vi "RTS Post Client Setup Data.vi"(8 "Error In":errorcluster, 10 "File Setup Data":string[][](array[string]), 11 "Station Settings In":T1) -> (0 "Error Out":errorcluster, 3 "Station Settings Out":T1)   [LabVIEW 2016]
uses:
  Type Definitions/RTS Station Settions TCP Comms.ctl
  Type Definitions/RTS Chamber Save Status.ctl
  Type Definitions/RTS Test Pattern.ctl
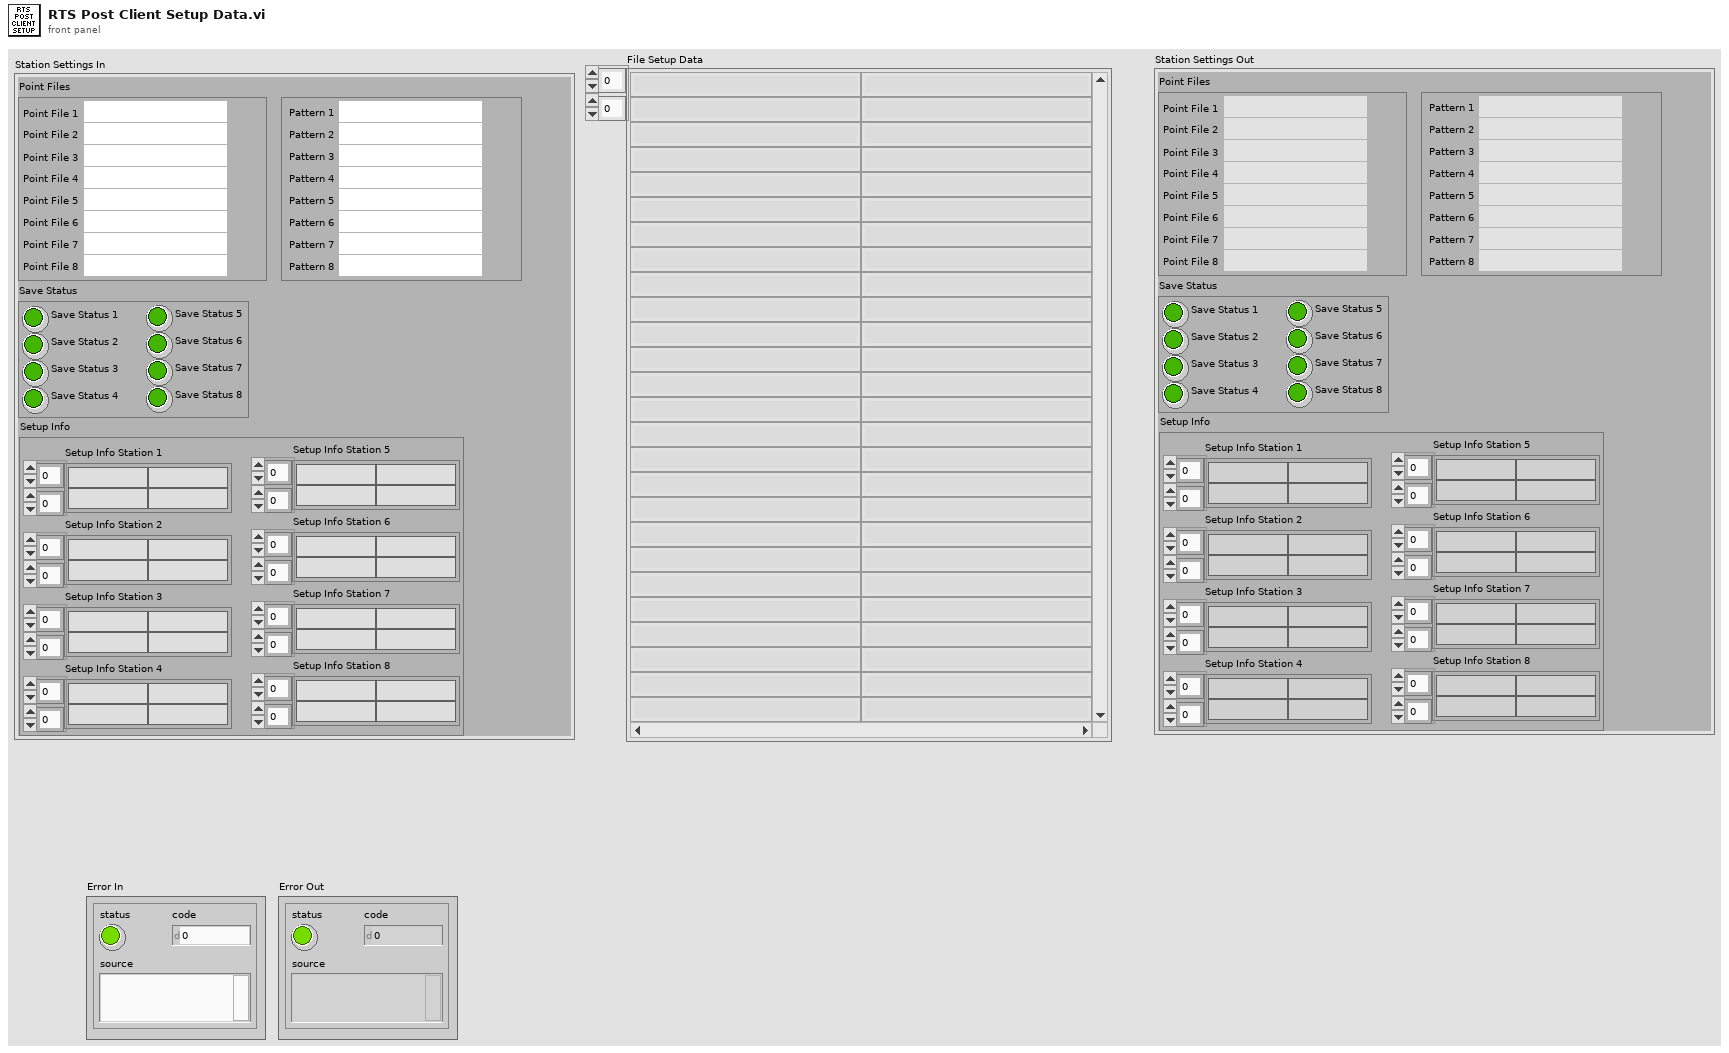
[diagram p1: front panel]
types:
  T1 = typedef "RTS Station Settions TCP Comms.ctl" = cluster{"Point Files":cluster{"Point File 1":path, "Point File 2":path, "Point File 3":path, "Point File 4":path, "Point File 5":path, "Point File 6":path, "Point File 7":path, "Point File 8":path}, "Save Status":T2, "Setup Info":cluster{"Setup Info Station 1":string[][], "Setup Info Station 2":string[][], "Setup Info Station 3":string[][], "Setup Info Station 4":string[][], "Setup Info Station 5":string[][], "Setup Info Station 6":string[][], "Setup Info Station 7":string[][], "Setup Info Station 8":string[][]}, "Chamber Test Pattern":T3}
  T2 = typedef "RTS Chamber Save Status.ctl" = cluster{"Save Status 1":bool, "Save Status 2":bool, "Save Status 3":bool, "Save Status 4":bool, "Save Status 5":bool, "Save Status 6":bool, "Save Status 7":bool, "Save Status 8":bool}
  T3 = typedef "RTS Test Pattern.ctl" = cluster{" Pattern 1":path, "Pattern 2":path, "Pattern 3":path, "Pattern 4":path, "Pattern 5":path, "Pattern 6":path, "Pattern 7":path, "Pattern 8":path}
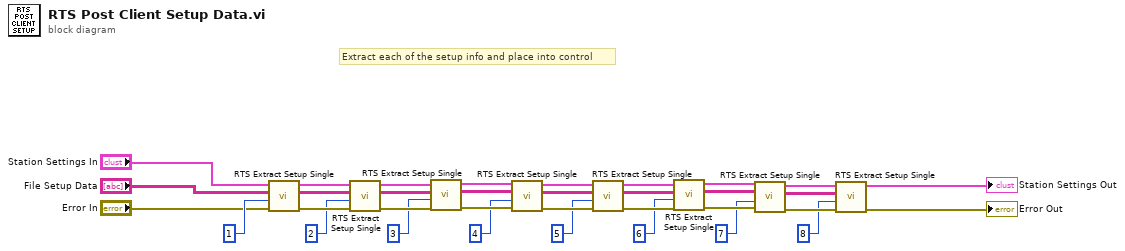
[diagram p0: block diagram]
diagram:
  # "Extract each of the setup info and place into control"
  n1 = call "RTS Extract Setup Single.vi"("Error In"="Error In", "Station Number"=u8 1, "File Setup Data"="File Setup Data", "Station Settings In in"="Station Settings In") -> ("Error Out"=w29:errorcluster, "Updated Array"=w31:string[][], "Station Settings In out"=w30:T1)  [unwired: 5 in]
  n2 = call "RTS Extract Setup Single.vi"("Error In"=w29, "Station Number"=u8 2, "File Setup Data"=w31, "Station Settings In in"=w30) -> ("Error Out"=w28:errorcluster, "Updated Array"=w22:string[][], "Station Settings In out"=w15:T1)  [unwired: 5 in]
  n3 = call "RTS Extract Setup Single.vi"("Error In"=w28, "Station Number"=u8 3, "File Setup Data"=w22, "Station Settings In in"=w15) -> ("Error Out"=w27:errorcluster, "Updated Array"=w21:string[][], "Station Settings In out"=w14:T1)  [unwired: 5 in]
  n4 = call "RTS Extract Setup Single.vi"("Error In"=w27, "Station Number"=u8 4, "File Setup Data"=w21, "Station Settings In in"=w14) -> ("Error Out"=w26:errorcluster, "Updated Array"=w20:string[][], "Station Settings In out"=w13:T1)  [unwired: 5 in]
  n5 = call "RTS Extract Setup Single.vi"("Error In"=w26, "Station Number"=u8 5, "File Setup Data"=w20, "Station Settings In in"=w13) -> ("Error Out"=w25:errorcluster, "Updated Array"=w19:string[][], "Station Settings In out"=w12:T1)  [unwired: 5 in]
  n6 = call "RTS Extract Setup Single.vi"("Error In"=w25, "Station Number"=u8 6, "File Setup Data"=w19, "Station Settings In in"=w12) -> ("Error Out"=w24:errorcluster, "Updated Array"=w18:string[][], "Station Settings In out"=w11:T1)  [unwired: 5 in]
  n7 = call "RTS Extract Setup Single.vi"("Error In"=w24, "Station Number"=u8 7, "File Setup Data"=w18, "Station Settings In in"=w11) -> ("Error Out"=w23:errorcluster, "Updated Array"=w17:string[][], "Station Settings In out"=w10:T1)  [unwired: 5 in]
  n8 = call "RTS Extract Setup Single.vi"("Error In"=w23, "Station Number"=u8 8, "File Setup Data"=w17, "Station Settings In in"=w10) -> ("Error Out"=→"Error Out":errorcluster, "Station Settings In out"=→"Station Settings Out":T1)  [unwired: 5 in, 1 out]
